vi "0624.vi"() -> ()   [LabVIEW 2013]
uses:
  <vilib>/Instr/_visa.llb/VISA Configure Serial Port (Instr).vi
panel:
  out "error out":errorcluster
  in  "stop":bool
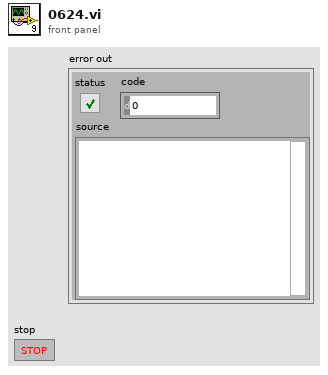
[diagram p1: front panel]
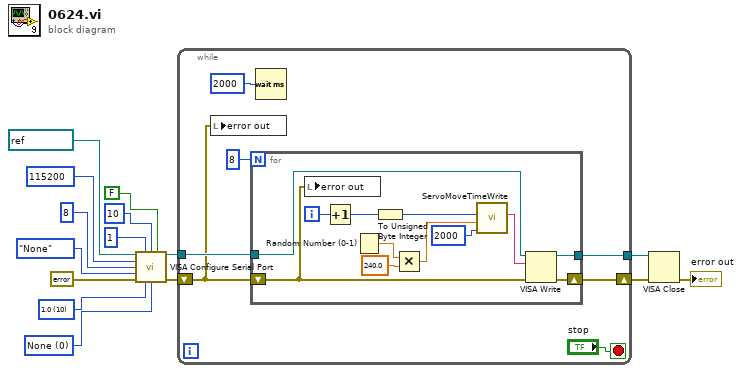
[diagram p0: block diagram]
diagram:
  w10 = u16 0 items=["None", "XON/XOFF", "RTS/CTS", "XON/XOFF & RTS/CTS", "DTR/DSR", "XON/XOFF & DTR/DSR"] ("flow control (0:none)")
  w11 = u16 10 items=["1.0"=10, "1.5"=15, "2.0"=20] ("stop bits (10: 1 bit)")
  n1 = call-poly "VISA Configure Serial Port"("VISA resource name"=refnum<visa-resource-name> "COM7", "timeout (10sec)"=u32 1, "termination char\n(0xA = '\\n' = LF)"=u8 10 ("termination char\n(0xA = '\\n' = LF)"), "Enable Termination\nChar (T)"=FALSE ("Enable Termination\nChar (T)"), "baud rate (9600)"=u32 115200, "data bits (8)"=u16 8, "parity (0:none)"=enum16{"None", "Odd", "Even", "Mark", "Space"}."None", "error in (no error)"=errorcluster {"status"=FALSE, "code"=0, "source"=""}, "stop bits (10: 1 bit)"=w11, "flow control (0:none)"=w10) -> ("VISA resource name out"=w5:refnum<visa-resource-name>, "error out"=w4:errorcluster)  [unwired: 4 in]
  n2 = while {
    tunnel: w5 -> [w20]
    shift-right: [w19] -> w3
    shift-left: w4 -> [w16]
    tunnel: [w18] -> w2
    stop <- "stop" stop-if-true
    n3 = local write "error out"(w16) -> ()
    n4 = for {
      N: 8 -> [_]
      shift-right: [w29] -> w19
      shift-left: w16 -> [w27]
      tunnel: w20 -> [w30]
      tunnel: [w28] -> w18
      i -> [w34]
      n5 = local write "error out"(w27) -> ()
      n6 = Increment(x=w34) -> (x+1=w32:i32)
      n7 = Random Number (0-1)() -> (number: 0 to 1=w26:dbl)
      n8 = To Unsigned Byte Integer(number=w32) -> (unsigned 8bit integer=w33:u8)
      n9 = Multiply(x=w26, y=240.0) -> (x*y=w24:dbl)
      n10 = call "ServoMoveTimeWrite.vi"("Time"=u16 2000 ("milliseconds to wait"), "Angel"=w24, "ID"=w33) -> ("Command"=w31:string)  [unwired: 8 in]
      n11 = VISA Write(VISA resource name=w30, write buffer=w31, error in (no error)=w27) -> (VISA resource name out=w28:refnum<visa-resource-name>, error out=w29:errorcluster)  [unwired: 1 out]
    }
    n12 = Wait (ms)(milliseconds to wait=u32 2000) -> ()  [unwired: 1 out]
  }
  n13 = VISA Close(VISA resource name=w2, error in (no error)=w3) -> (error out=→"error out":errorcluster)
